vi "MARS Read TDMS Scan Data.vi"(10 "Active Meas.":i32, 11 "Listbox":i32[](array[numeric])) -> (0 "Scan Total Int":i32[][](array[numeric]), 3 "Scan Tail Int":i32[][](array[numeric]), 4 "FoM_2nd_max":dbl, 5 "FoM_1st_max":dbl, 6 "FoM_2nd_min":dbl, 7 "FoM_1st_min":dbl)   [LabVIEW 2015]
uses:
  Data_Analysis_subvis/ESA_Data_Analysis_Global_VIs.vi
  Data_Analysis_subvis/MARS_Scan_Data_Analysis_global.vi
panel:
  out "subarray":string[](array[string])
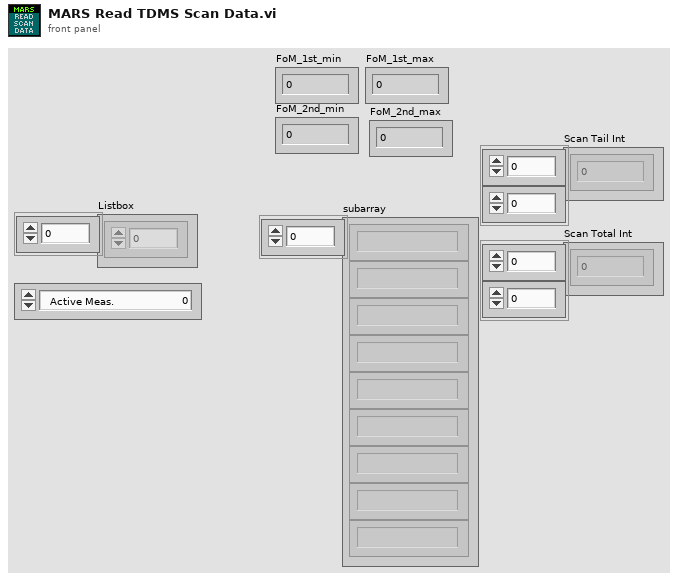
[diagram p1: front panel]
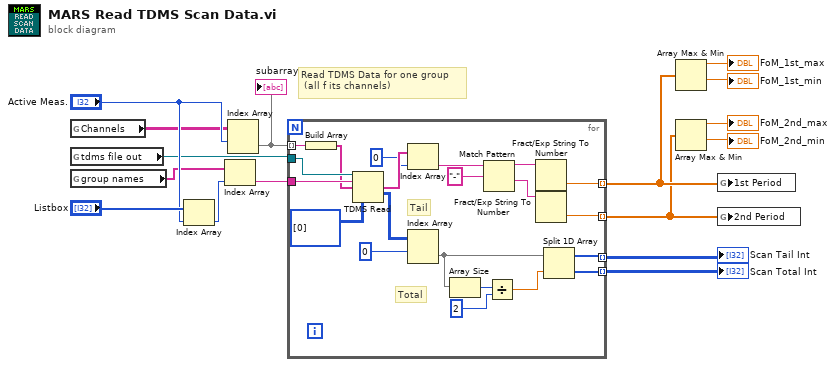
[diagram p0: block diagram]
diagram:
  # "Read TDMS Data for one group\n (all f its channels)"
  n1 = global read "MARS_Scan_Data_Analysis_global.vi" "Channels"() -> (w9:string[][])
  n2 = global read "ESA_Data_Analysis_Global_VIs.vi" "tdms file out"() -> (w7:refnum<k34>)
  n3 = global read "ESA_Data_Analysis_Global_VIs.vi" "group names"() -> (w8:string[])
  n4 = Index Array(array="Listbox", index="Active Meas.") -> (element=w14:i32)
  n5 = Index Array(array=w8, index=w14) -> (element=w12:string)
  n6 = Index Array(array=w9, index (row)="Active Meas.") -> (element=w13:string[])  [unwired: 1 in]
  "subarray" <- w13
  n7 = for {
    tunnel: w7 -> [w37]
    tunnel: w12 -> [w36]
    tunnel: w13 -> [w33] mode=indexing
    tunnel: [w25] -> w6 mode=indexing
    tunnel: [w24] -> w5 mode=indexing
    tunnel: [w19] -> w15 mode=indexing
    tunnel: [w18] -> w16 mode=indexing
    # "Total"
    # "Tail"
    n8 = Build Array(w33) -> (w32:string[])
    n9 = TDMS Read(0:w37, 5:w36, 7:w32, 12:i32[][] [[0]] ("unsigned byte array")) -> (8:w28:string[], 10:w34:i32[][])  [unwired: 4 in, 4 out]
    n10 = Index Array(array=w28, index=0) -> (element=w26:string)
    n11 = Index Array(array=w34, index (row)=0) -> (element=w22:i32[])  [unwired: 1 in]
    n12 = Array Size(array=w22) -> (size(s)=w21:i32)
    n13 = Match Pattern(string=w26, regular expression="-") -> (before substring=w30:string, after substring=w31:string)  [unwired: 1 in, 2 out]
    n14 = Divide(x=w21, y=2) -> (x/y=w17:dbl)
    n15 = Fract/Exp String To Number(string=w30) -> (number=w25:dbl)  [unwired: 3 in, 1 out]
    n16 = Fract/Exp String To Number(string=w31) -> (number=w24:dbl)  [unwired: 3 in, 1 out]
    n17 = Split 1D Array(array=w22, index=w17) -> (first subarray=w19:i32[], second subarray=w18:i32[])
  }
  "Scan Tail Int" <- w15
  "Scan Total Int" <- w16
  n18 = Array Max & Min(array=w6) -> (max value=→"FoM_1st_max":dbl, min value=→"FoM_1st_min":dbl)  [unwired: 2 out]
  n19 = Array Max & Min(array=w5) -> (max value=→"FoM_2nd_max":dbl, min value=→"FoM_2nd_min":dbl)  [unwired: 2 out]
  n20 = global write "MARS_Scan_Data_Analysis_global.vi" "1st Period"(w6) -> ()
  n21 = global write "MARS_Scan_Data_Analysis_global.vi" "2nd Period"(w5) -> ()
